vi "GoToKick.vi"(1 "goleiro?":bool, 3 "balls":T3[](array[typedef]), 4 "Robot in in":T4, 5 "atacando contra?":bool, 6 "Field Size in":T2, 7 "Target":dbl[](array[numeric]), 8 "Defender":bool, 9 "D ball - robot":dbl, 10 "AI Parameters":T1={"GotoKick"={"Dist do cone a frente"=150.0, "attacker farback"=1500.0, "Perto"=300.0, "min dist to kick"=150.0, "kick eps"=0.05, "Time to transition"=0.0}, "Attacker"={"CC chute"=0.09, "CC passe"=0.045, "Kick Force"=100.0, "D ball-robot Kick"=200.0, "D ball-robot Pass"=0.3}, "Defender"={"D max"=1700.0, "Vel p/ robô av"=1000.0, "Kick Force"=100.0, "D atk-def"=0.0, "D farback"=0.0}, "Timeout"={"Field/v in x"=6.0, "Dist Robots"=300, "Dist up in y"=300}, "Pose Striker"={"dist"=200.0, "Numeric"=-4.0, "dist 2"=200.0}, "Dist Stop"=300.0, "Distance when ball out"=200, "D central gap "=150.0, "T pass"=0.0, "Force ++"=0.0, "range kick"=0.0, "Chute alto"=TRUE, "Marcador novo"=TRUE} {"D central gap" format="%#_13g"; "Dist Stop" format="%#_13g"; "Pose Striker"."Numeric" format="%#_13g"; "Defender"."Kick Force" format="%#_13g"; "Defender"."Vel p/ robô av" format="%#_13g"; "Attacker"."D ball-robot Kick" format="%#_13g"; "Attacker"."Kick Force" format="%#_13g"; "Attacker"."CC passe" format="%#_13g"; "Attacker"."CC chute" format="%#_13g"; "GotoKick"."kick eps" format="%#_13g"; "GotoKick"."min dist to kick" format="%#_13g"; "GotoKick"."Perto" format="%#_13g"; "GotoKick"."attacker farback" format="%#_13g"; "GotoKick"."Dist do cone a frente" format="%#_13g"}, 11 "Cone de chute":dbl=0.09 format="%#_13g", 13 "Passe":bool, 18 "Kick Force":dbl=5.0 format="%#_13g", 19 "IA State Input in":T7) -> (0 "Current States":T6, 12 "Next State":T6, 14 "Robot out":T4, 17 "kick error":dbl)   [LabVIEW 2017]
uses:
  Core/AI Input.ctl
  Core/AI Robot.ctl
  Functions Enum.ctl
  AttackerStates.ctl
  Core/AI Ball.ctl
  Core/Field Size.ctl
  Core/AI Judge.ctl
  Command Enum.ctl
  Util/Events/Events.ctl
  AI Parameters.ctl
  <vilib>/Analysis/_algsub.llb/Real Vector Norm.vi
  <vilib>/Analysis/baseanly.llb/Real Dot Product.vi
  <vilib>/Analysis/coordinate.llb/2D Cartesian Coordinate Rotation (Scalar).vi
  <vilib>/Analysis/NI_AALPro.lvlib
  <vilib>/Analysis/NI_AALBase.lvlib
panel:
  out "Elapsed Time (s)":dbl
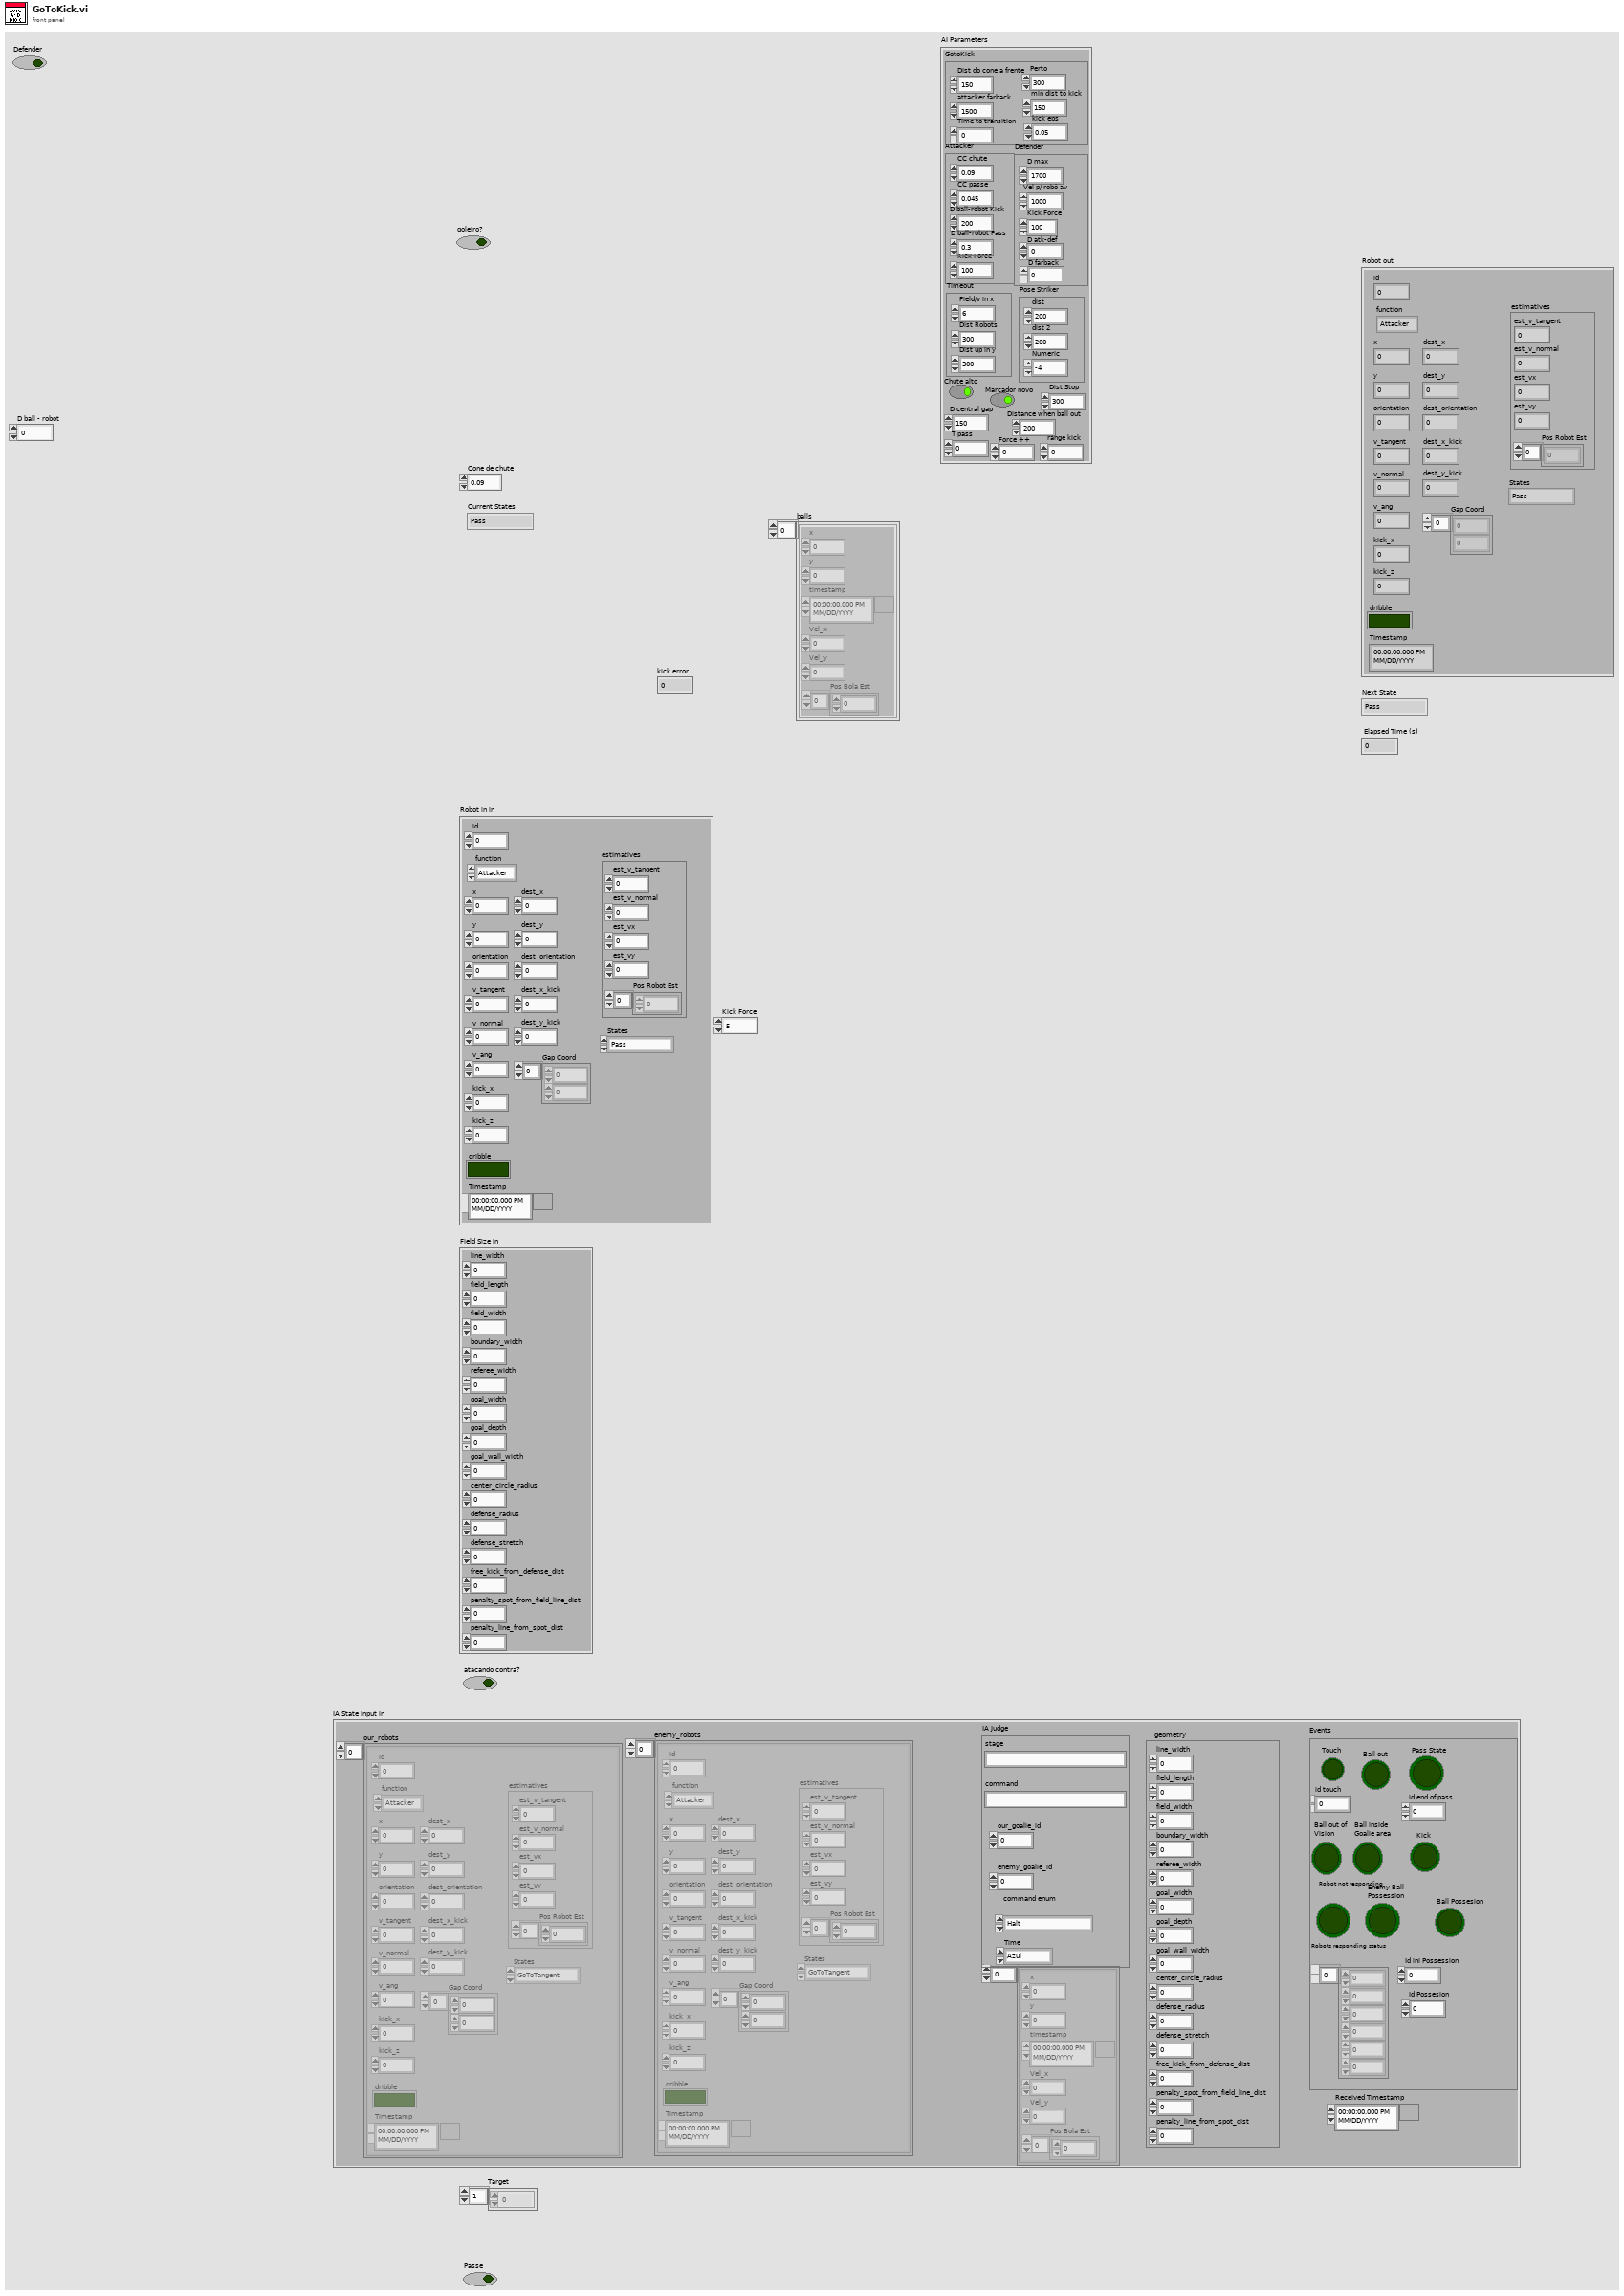
[diagram p1: front panel]
types:
  T1 = typedef "AI Parameters.ctl" = cluster{"GotoKick":cluster{"Dist do cone a frente":dbl, "attacker farback":dbl, "Perto":dbl, "min dist to kick":dbl, "kick eps":dbl, "Time to transition":dbl}, "Attacker":cluster{"CC chute":dbl, "CC passe":dbl, "Kick Force":dbl, "D ball-robot Kick":dbl, "D ball-robot Pass":dbl}, "Defender":cluster{"D max":dbl, "Vel p/ robô av":dbl, "Kick Force":dbl, "D atk-def":dbl, "D farback":dbl}, "Timeout":cluster{"Field/v in x":dbl, "Dist Robots":u32, "Dist up in y":u32}, "Pose Striker":cluster{"dist":dbl, "Numeric":dbl, "dist 2":dbl}, "Dist Stop":dbl, "Distance when ball out":i32, "D central gap ":dbl, "T pass":dbl, "Force ++":dbl, "range kick":dbl, "Chute alto":bool, "Marcador novo":bool}
  T2 = typedef "Field Size.ctl" = cluster{"line_width":u32, "field_length":u32, "field_width":u32, "boundary_width":u32, "referee_width":u32, "goal_width":u32, "goal_depth":u32, "goal_wall_width":u32, "center_circle_radius":u32, "defense_radius":u32, "defense_stretch":u32, "free_kick_from_defense_dist":u32, "penalty_spot_from_field_line_dist":u32, "penalty_line_from_spot_dist":u32}
  T3 = typedef "AI Ball.ctl" = cluster{"x":dbl, "y":dbl, "timestamp":timestamp, "Vel_x":dbl, "Vel_y":dbl, "Pos Bola Est":dbl[]}
  T4 = typedef "AI Robot.ctl" = cluster{"id":u32, "function":T5, "x":dbl, "y":dbl, "orientation":dbl, "v_tangent":dbl, "v_normal":dbl, "v_ang":dbl, "kick_x":dbl, "kick_z":dbl, "dribble":bool, "Timestamp":timestamp, "dest_x":dbl, "dest_y":dbl, "dest_orientation":dbl, "estimatives":cluster{"est_v_tangent":dbl, "est_v_normal":dbl, "est_vx":dbl, "est_vy":dbl, "Pos Robot Est":dbl[]}, "dest_x_kick":dbl, "dest_y_kick":dbl, "Gap Coord":dbl[], "States":T6}
  T5 = typedef "Functions Enum.ctl" = enum16{"Attacker", "Goalie", "Defender", "Striker", "Goto 0", "Dummy", "Kicker", "ZigZag"}
  T6 = typedef "AttackerStates.ctl" = enum16{"Pass", "GoToTangent", "BallGetting", "GoToKick", ""}
  T7 = typedef "AI Input.ctl" = cluster{"our_robots":T4[], "enemy_robots":T4[], "balls":T3[], "geometry":T2, "IA Judge":T8, "Received Timestamp":timestamp, "Events":T10}
  T8 = typedef "AI Judge.ctl" = cluster{"stage":string, "command":string, "our_goalie_id":dbl, "enemy_goalie_id":dbl, "command enum":T9, "Time":enum16{"Azul", "Amarelo"}}
  T9 = typedef "Command Enum.ctl" = enum16{"Halt", "Stop", "Force Start", "PKA Normal Start", "Prepare Kickoff Ally", "PKE Normal Start", "Prepare Kickoff Enemy", "Prepare Penalty Ally", "PPA Normal Start", "Prepare Penalty Enemy", "PPE Normal Start", "Direct Free Enemy", "Direct Free Ally", "Indirect Free Enemy", "Indirect Free Ally", "Timeout Enemy", "Timeout Ally", "Goal Enemy", "Goal Ally", "Ball Placement Enemy", "Ball Placement Ally", "Normal Half Time", "Extra Time Break", "Extra Half Time", "None", "Post Game"}
  T10 = typedef "Events.ctl" = cluster{"Touch":bool, "Ball out":bool, "id touch":dbl, "Ball out of \nVision":bool, "Ball inside \nGoalie area":bool, "Robot not responding":bool, "Robots responding status":dbl[], "Enemy Ball \nPossession":bool, "Pass State":bool, "id end of pass":dbl, "Kick":bool, "Id ini Possession":dbl, "Ball Possesion":bool, "Id Possesion":dbl}
  T11 = cluster{"Dist do cone a frente":dbl, "attacker farback":dbl, "Perto":dbl, "min dist to kick":dbl, "kick eps":dbl, "Time to transition":dbl}
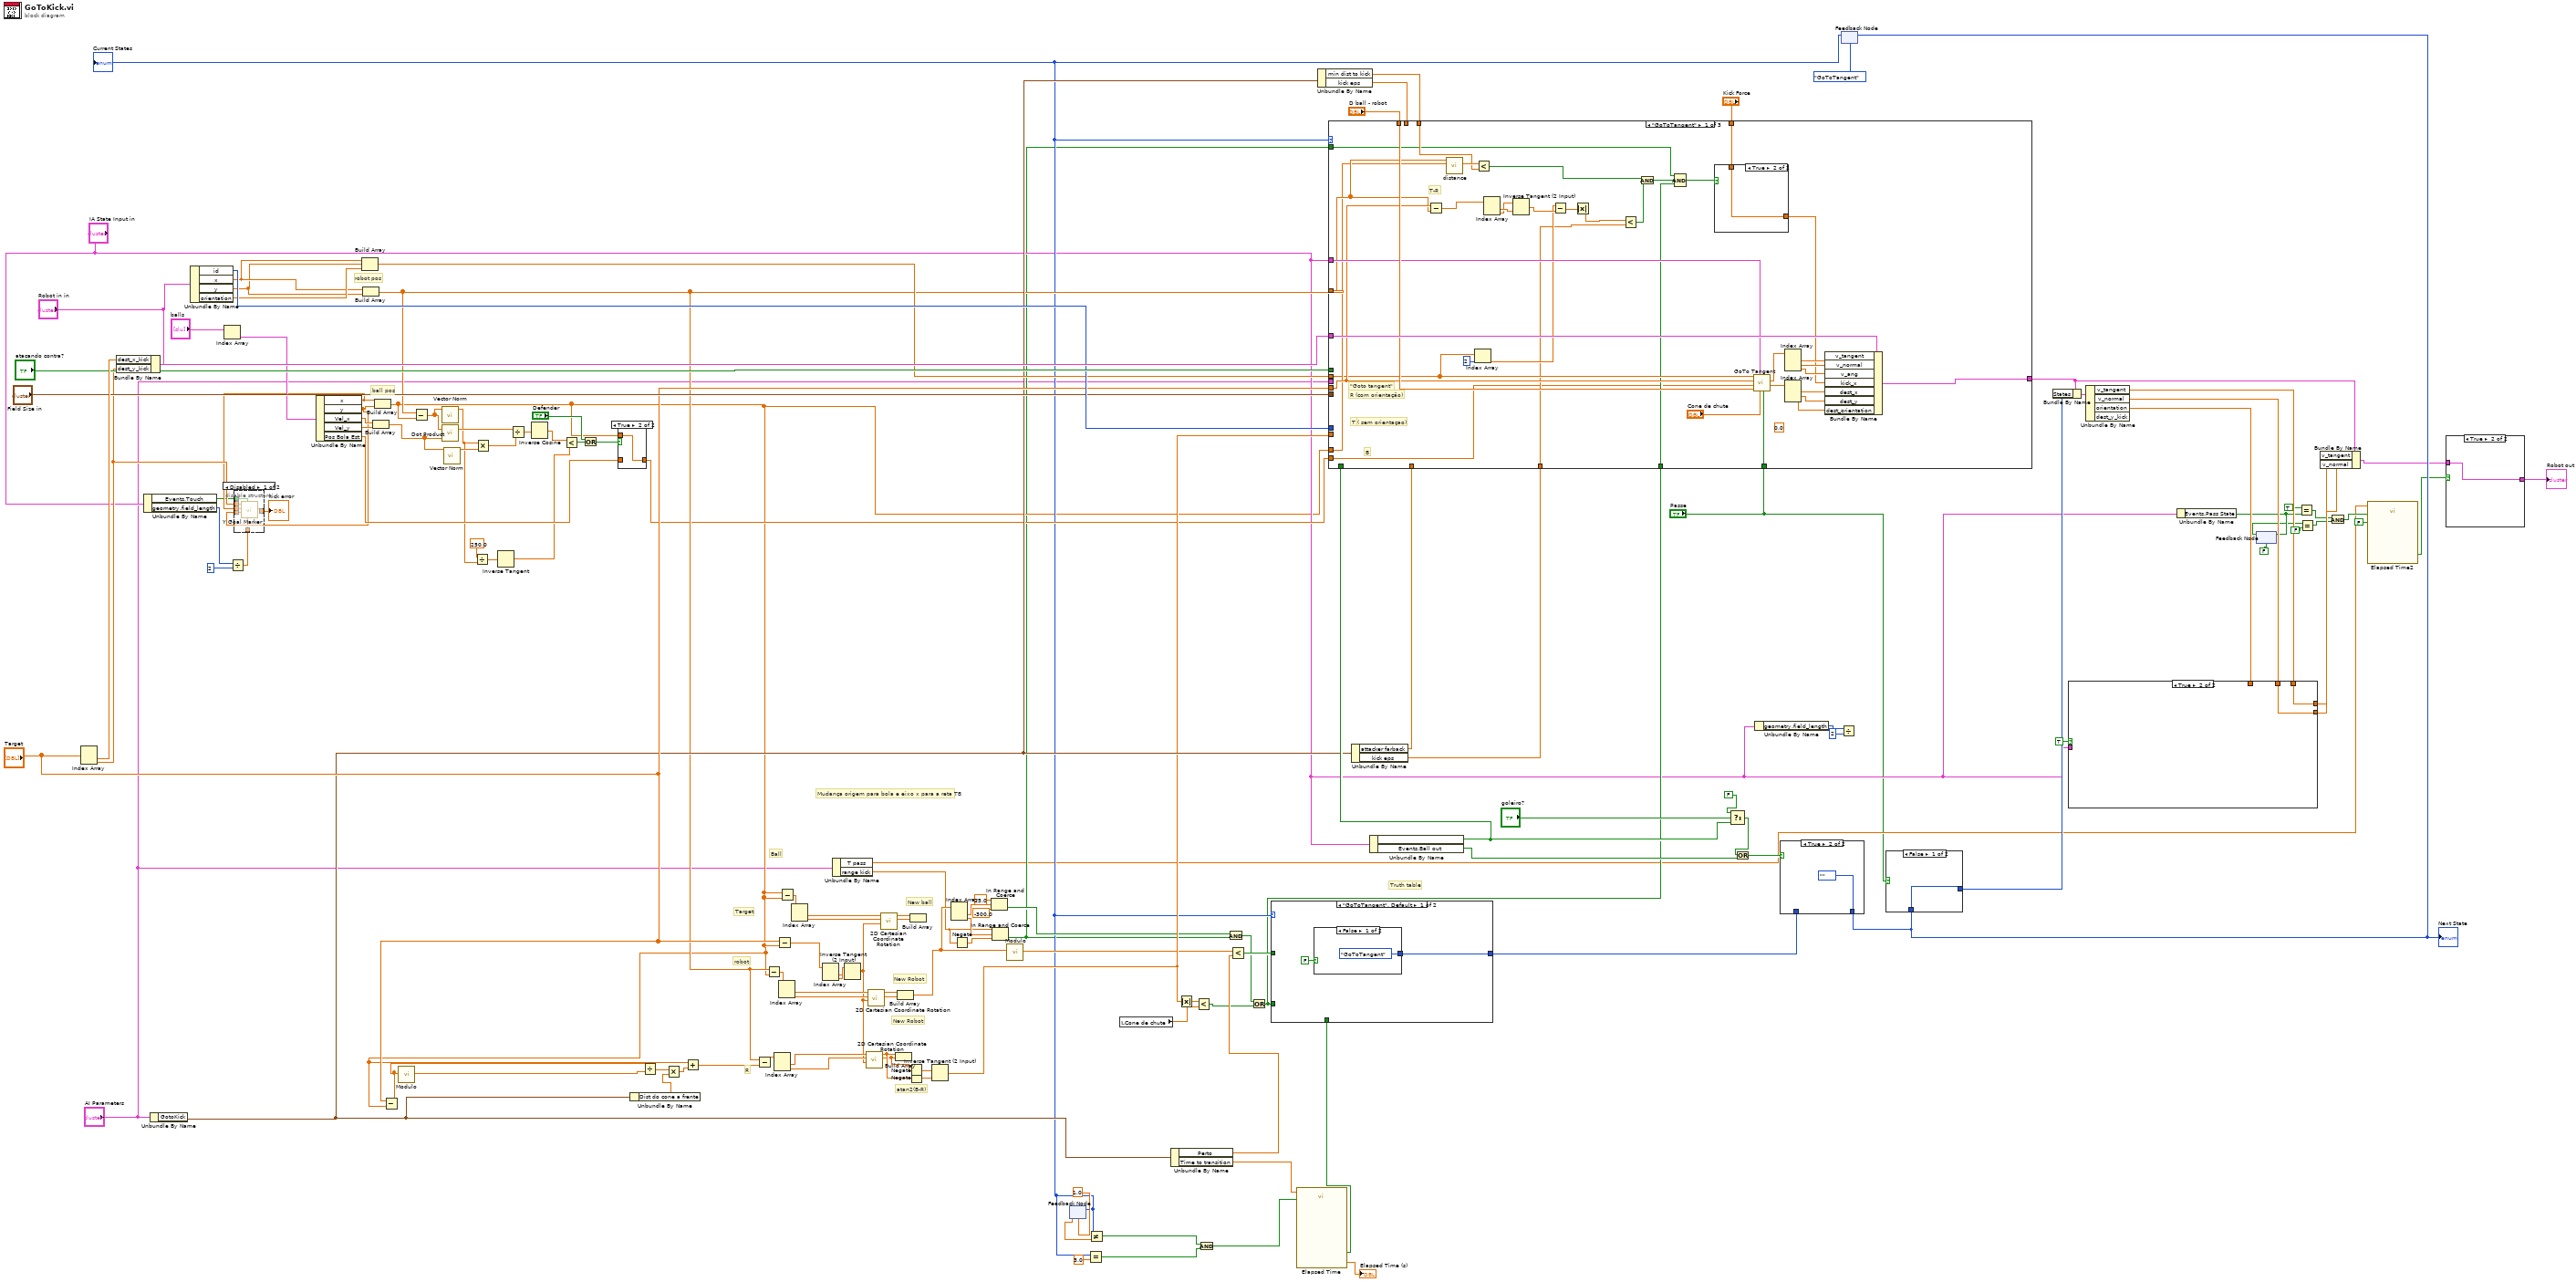
[diagram p0: block diagram]
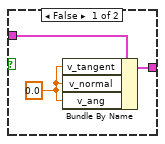
[diagram p3: hidden frame]
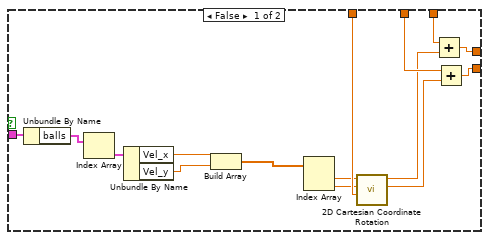
[diagram p4: hidden frame]
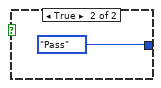
[diagram p6: hidden frame]
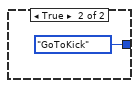
[diagram p7: hidden frame]
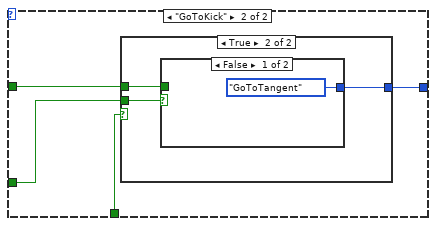
[diagram p8: hidden frame]
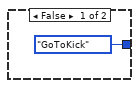
[diagram p9: hidden frame]
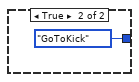
[diagram p10: hidden frame]
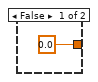
[diagram p12: hidden frame]
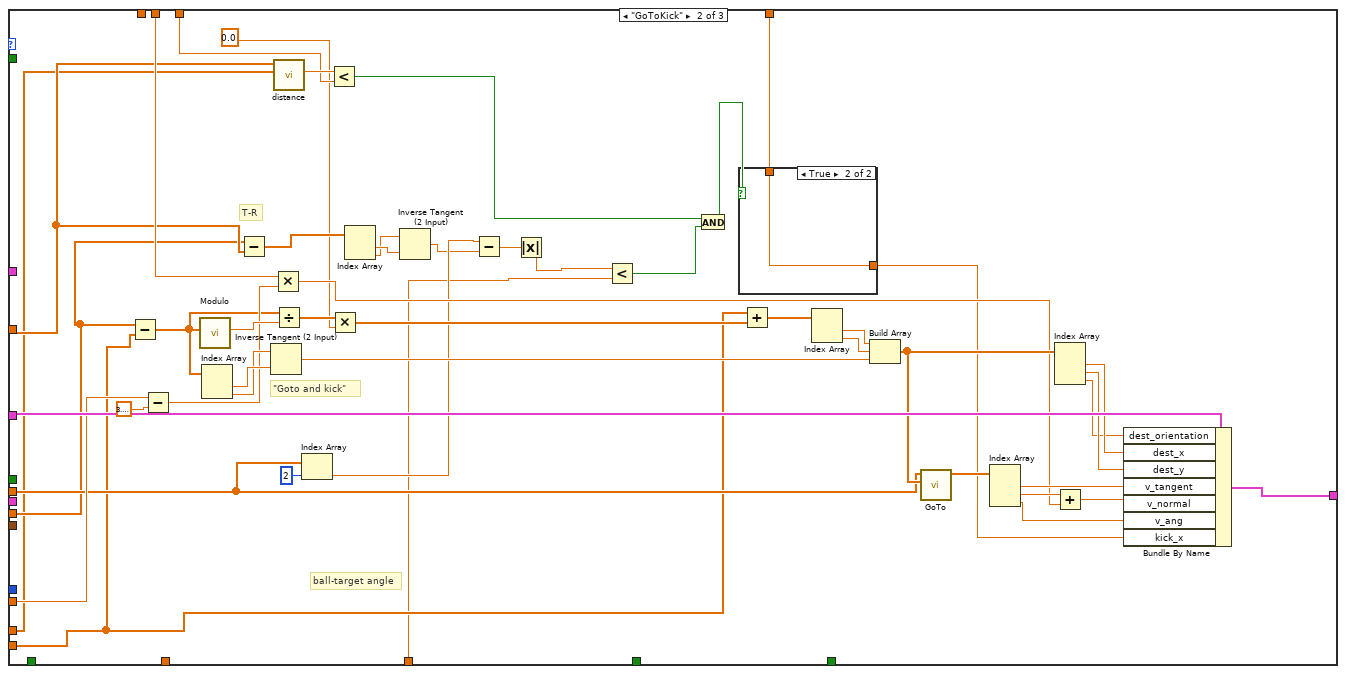
[diagram p13: hidden frame]
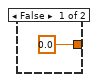
[diagram p14: hidden frame]
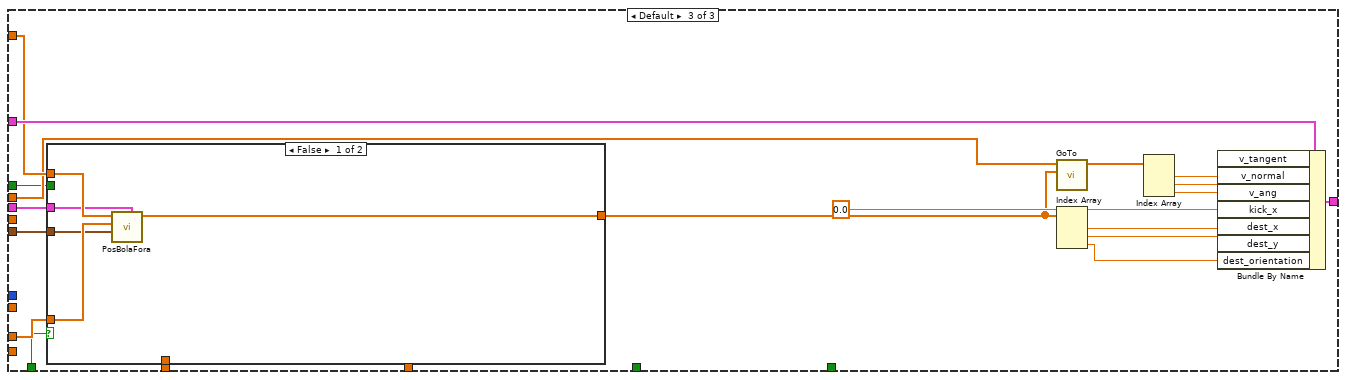
[diagram p15: hidden frame]
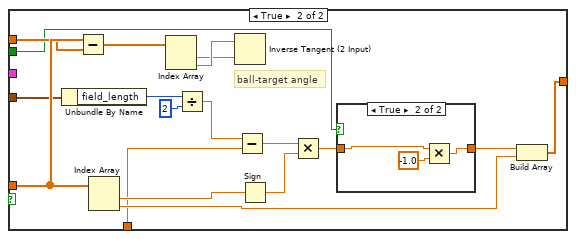
[diagram p16: hidden frame]
diagram:
  # "New ball"
  # "robot"
  # "atan2(B-R)"
  # "New Robot"
  # "New Robot"
  # "R"
  # "Ball"
  # "Target"
  # "Mudança origem para bola e eixo x para a reta TB"
  # "Truth table"
  # "robot pos"
  # "ball pos"
  n1 = Index Array(array="Target") -> (element #1=w139:dbl, element #2=w34:dbl)  [unwired: 2 in]
  n2 = Bundle By Name(cluster="Robot in in", "dest_x_kick"=w139, "dest_y_kick"=w34) -> (w135:T4)
  n3 = Unbundle By Name("IA State Input in") -> ("Events.Touch"=w30:bool, "geometry.field_length"=w29:u32)
  n4 = Unbundle By Name("AI Parameters") -> ("GotoKick"=w80:T11)
  n5 = Unbundle By Name("Robot in in") -> ("id"=w110:u32, "x"=w74:dbl, "y"=w73:dbl, "orientation"=w101:dbl)
  n6 = Index Array(array="balls") -> (element=w99:T3)  [unwired: 1 in]
  n7 = Divide(x=w29, y=u32 2) -> (x/y=w27:dbl)
  n8 = Unbundle By Name(w99) -> ("x"=w33:dbl, "y"=w32:dbl, "Vel_x"=w56:dbl, "Vel_y"=w55:dbl, "Pos Bola Est"=w47:dbl[])
  n9 = disable-structure shown="Disabled" {
    disable-tunnel: w34 -> [w145 _]
    disable-tunnel: w33 -> [w144 _]
    disable-tunnel: w32 -> [w143 _]
    disable-tunnel: w30 -> [w142 _]
    disable-tunnel: w27 -> [w141 _]
    disable-tunnel: [w140 _] -> w26
    frame Disabled {
      n10 = call "Y Goal Marker.vi"("goal x"=w141, "Touch"=w142, "ball y"=w143, "ball x"=w144, "dest_y_kick"=w145) -> ("kick error"=w140:dbl)  [unwired: 5 in, 1 out]
    }
    frame Enabled {
    }
  }
  "kick error" <- w26
  n11 = Build Array(w74, w73, w101) -> (w100:dbl[])
  n12 = Build Array(w74, w73) -> (w57:dbl[])
  n13 = Build Array(w56, w55) -> (w53:dbl[])
  n14 = Build Array(w33, w32) -> (w20:dbl[])
  n15 = Subtract(x="Target", y=w20) -> (x-y=w129:dbl[])
  n16 = call "Modulo.vi"("2D vector"=w129) -> ("Modulo"=w128:dbl)  [unwired: 10 in]
  n17 = Subtract(x=w57, y=w20) -> (x-y=w54:dbl[])
  n18 = call-poly <vilib>:"Dot Product.vi"("Y Vector"=w53, "X Vector"=w54) -> ("X * Y"=w50:dbl)  [unwired: 1 out]
  n19 = call-poly <vilib>:"Vector Norm.vi"("Input Vector"=w54) -> ("norm"=w44:dbl)  [unwired: 9 in, 1 out]
  n20 = call-poly <vilib>:"Vector Norm.vi"("Input Vector"=w53) -> ("norm"=w52:dbl)  [unwired: 9 in, 1 out]
  n21 = Divide(x=250.0, y=w44) -> (x/y=w45:dbl)
  n22 = Multiply(x=w44, y=w52) -> (x*y=w51:dbl)
  n23 = Inverse Tangent(1:w45) -> (0:w42:dbl)
  n24 = Divide(x=w50, y=w51) -> (x/y=w49:dbl)
  n25 = Inverse Cosine(1:w49) -> (0:w48:dbl)
  n26 = Less?(x=w48, y=w42) -> (x < y?=w22:bool)
  n27 = Or(x="Defender", y=w22) -> (x .or. y?=w23:bool)
  n28 = case shown="True" w23 {
    tunnel: w47 -> [w146 _]
    tunnel: [w146 w147] -> w46
    tunnel: w20 -> [_ w147]
    frame False {
    }
    frame True {
    }
  }
  n29 = Unbundle By Name(w80) -> ("Dist do cone a frente"=w86:dbl)
  n30 = Divide(x=w129, y=w128) -> (x/y=w127:dbl[])
  n31 = Multiply(x=w127, y=w86) -> (x*y=w126:dbl[])
  n32 = Add(x=w20, y=w126) -> (x+y=w130:dbl[])
  n33 = Subtract(x=w57, y=w130) -> (x-y=w131:dbl[])
  n34 = Subtract(x=w57, y=w20) -> (x-y=w104:dbl[])
  n35 = Index Array(array=w131) -> (element #1=w132:dbl, element #2=w133:dbl)  [unwired: 2 in]
  n36 = Subtract(x="Target", y=w20) -> (x-y=w105:dbl[])
  n37 = Index Array(array=w104) -> (element #1=w102:dbl, element #2=w103:dbl)  [unwired: 2 in]
  n38 = Subtract(x=w20, y=w20) -> (x-y=w70:dbl[])
  n39 = Index Array(array=w70) -> (element #1=w68:dbl, element #2=w69:dbl)  [unwired: 2 in]
  n40 = Index Array(array=w105) -> (element #1=w106:dbl, element #2=w107:dbl)  [unwired: 2 in]
  n41 = Unbundle By Name("AI Parameters") -> ("T pass"=w2:dbl, "range kick"=w3:dbl)
  n42 = Inverse Tangent (2 Input)(1:w106, 2:w107) -> (0:w67:dbl)
  n43 = call-poly <vilib>:"2D Cartesian Coordinate Rotation.vi"("theta"=w67, "y"=w133, "x"=w132) -> ("y out"=w124:dbl, "x out"=w125:dbl)  [unwired: 6 in, 1 out]
  n44 = call-poly <vilib>:"2D Cartesian Coordinate Rotation.vi"("theta"=w67, "y"=w103, "x"=w102) -> ("y out"=w109:dbl, "x out"=w66:dbl)  [unwired: 6 in, 1 out]
  n45 = call-poly <vilib>:"2D Cartesian Coordinate Rotation.vi"("theta"=w67, "y"=w69, "x"=w68) -> ("y out"=w71:dbl, "x out"=w72:dbl)  [unwired: 6 in, 1 out]
  n46 = Build Array(w125, w124) -> ()  [unwired: 1 out]
  n47 = Build Array(w66, w109) -> (w65:dbl[])
  n48 = Negate(x=w124) -> (-x=w122:dbl)
  n49 = Negate(x=w125) -> (-x=w123:dbl)
  n50 = Build Array(w72, w71) -> ()  [unwired: 1 out]
  n51 = Inverse Tangent (2 Input)(1:w123, 2:w122) -> (0:w78:dbl)
  n52 = Index Array(array=w65) -> (element #1=w64:dbl, element #2=w63:dbl)  [unwired: 2 in]
  n53 = Negate(x=w3) -> (-x=w4:dbl)
  n54 = In Range and Coerce(upper limit=25.0, x=w64, lower limit=-300.0) -> (In Range?=w60:bool)  [unwired: 1 out]
  n55 = In Range and Coerce(upper limit=w3, x=w63, lower limit=w4) -> (In Range?=w6:bool)  [unwired: 1 out]
  n56 = call "Modulo.vi"("2D vector"=w65) -> ("Modulo"=w77:dbl)  [unwired: 10 in]
  n57 = feedback #1(1.0 ("Current State")) -> (w116:dbl)
  n58 = local read "Cone de chute"() -> (w25:dbl)
  n59 = Unbundle By Name(w80) -> ("Perto"=w76:dbl, "Time to transition"=w82:dbl)
  n60 = Absolute Value(x=w78) -> (abs(x)=w79:dbl)
  n61 = Less?(x=w79, y=w25) -> (x < y?=w59:bool)
  n62 = And(x=w60, y=w6) -> (x .and. y?=w58:bool)
  n63 = Less?(x=w77, y=w76) -> (x < y?=w75:bool)
  n64 = Or(x=w58, y=w59) -> (x .or. y?=w39:bool)
  n65 = Unbundle By Name(w80) -> ("min dist to kick"=w84:dbl, "kick eps"=w83:dbl)
  n66 = Unbundle By Name(w80) -> ("attacker farback"=w85:dbl, "kick eps"=w35:dbl)
  n67 = Unbundle By Name("IA State Input in") -> ("Events.Ball inside \nGoalie area"=w88:bool, "Events.Ball out"=w120:bool)
  n68 = Select(t=FALSE, s="goleiro?", f=w88) -> (s? t:f=w87:bool)
  n69 = Or(x=w87, y=w120) -> (x .or. y?=w121:bool)
  n70 = Unbundle By Name("IA State Input in") -> ("geometry.field_length"=w37:u32)
  n71 = Divide(x=w37, y=u32 2) -> ()  [unwired: 1 out]
  n72 = feedback #2(AttackerStates."GoToTangent" ("Next State")) -> (w41:T6)
  "Current States" <- w41
  n73 = feedback-in #1(w41) -> ()
  n74 = Equal?(x=w41, y=3.0) -> (x = y?=w113:bool)
  n75 = Not Equal?(x=w41, y=w116) -> (x != y?=w114:bool)
  n76 = And(x=w114, y=w113) -> (x .and. y?=w118:bool)
  n77 = call "Elapsed Time"("Time Target (s)"=w82, "Reset"=w118) -> ("Elapsed Time (s)"=→"Elapsed Time (s)":dbl, "Time has Elapsed"=w111:bool)  [unwired: 10 in, 6 out]
  n78 = case shown="\"GoToTangent\", Default" w41 {
    tunnel: [w149 w154] -> w136
    tunnel: w111 -> [_ w155]
    tunnel: w39 -> [_ w153]
    tunnel: w75 -> [_ w152]
    frame "GoToTangent", Default {
      n79 = case shown="False" FALSE {
        tunnel: [AttackerStates."GoToTangent" ("Next State") AttackerStates."GoToKick" ("Next State")] -> w149
        frame False {
        }
        frame True {
        }
      }
    }
    frame "GoToKick" {
      n80 = case shown="True" w155 {
        tunnel: [AttackerStates."GoToKick" ("Next State") w159] -> w154
        tunnel: w153 -> [_ w158]
        tunnel: w152 -> [_ w157]
        frame False {
        }
        frame True {
          n81 = case shown="False" w158 {
            tunnel: [AttackerStates."GoToTangent" ("Next State") AttackerStates."GoToKick" ("Next State")] -> w159
            tunnel: w157 -> [_ _]
            frame False {
            }
            frame True {
            }
          }
        }
      }
    }
  }
  n82 = case shown="\"GoToTangent\"" w41 {
    tunnel: [w191 w249 w270] -> w38
    tunnel: w135 -> [w192 w248 w269]
    tunnel: w100 -> [w172 w215 w263]
    tunnel: w57 -> [w176 w209 w265]
    tunnel: w20 -> [w175 w205 w266]
    tunnel: "Target" -> [w177 w208 _]
    tunnel: "Field Size in" -> [_ _ w264]
    tunnel: w110 -> [_ _ _]
    tunnel: w88 -> [_ _ w259]
    tunnel: "atacando contra?" -> [_ _ w258]
    tunnel: w78 -> [_ w229 _]
    tunnel: w85 -> [_ _ w253]
    tunnel: w84 -> [w174 w223 _]
    tunnel: w83 -> [_ w222 _]
    tunnel: "D ball - robot" -> [w189 _ _]
    tunnel: "AI Parameters" -> [_ _ w252]
    tunnel: "IA State Input in" -> [w188 _ _]
    tunnel: w46 -> [w164 w206 _]
    tunnel: "Kick Force" -> [w178 w204 _]
    tunnel: w39 -> [w168 _ _]
    tunnel: w35 -> [w166 w203 _]
    tunnel: w6 -> [w163 _ _]
    tunnel: "Passe" -> [w162 _ _]
    frame "GoToTangent" {
      (unwired) 0.0
      # "T-R"
      # "\"Goto tangent\""
      # "B"
      # "T"
      # "R ( sem orientaçao)"
      # "R (com orientação)"
      n83 = Subtract(x=w177, y=w176) -> (x-y=w184:dbl[])
      n84 = call "distance.vi"("target pos"=w175, "obj pos"=w176) -> ("sqrt(x)"=w187:dbl)  [unwired: 9 in]
      n85 = Index Array(array=w172, index=2) -> (element=w171:dbl)
      n86 = Less?(x=w187, y=w174) -> (x < y?=w183:bool)
      n87 = Index Array(array=w184) -> (element #1=w186:dbl, element #2=w185:dbl)  [unwired: 2 in]
      n88 = Inverse Tangent (2 Input)(1:w186, 2:w185) -> (0:w182:dbl)
      n89 = Subtract(x=w171, y=w182) -> (x-y=w181:dbl)
      n90 = Absolute Value(x=w181) -> (abs(x)=w179:dbl)
      n91 = Less?(x=w179, y=w166) -> (x < y?=w180:bool)
      n92 = And(x=w183, y=w180) -> (x .and. y?=w169:bool)
      n93 = Compound Arithmetic op=AND(w163, w169, w168) -> (w167:bool)
      n94 = case shown="True" w167 {
        tunnel: [0.0 w201] -> w170
        tunnel: w178 -> [_ w201]
        frame False {
        }
        frame True {
        }
      }
      n95 = call "GoTo Tangent.vi"("Passe"=w162, "Cone de chute"="Cone de chute", "IA State Input in"=w188, "distance between ball and robot"=w189, "Ball"=w164, "Target"=w177, "R"=w172) -> ("Destination"=w196:dbl[], "Output\nVelocity"=w197:dbl[])  [unwired: 3 in]
      n96 = Index Array(array=w197) -> (element #1=w199:dbl, element #2=w193:dbl, element #3=w198:dbl)  [unwired: 3 in]
      n97 = Index Array(array=w196) -> (element #1=w195:dbl, element #2=w194:dbl, element #3=w190:dbl)  [unwired: 3 in]
      n98 = Bundle By Name(cluster=w192, "v_tangent"=w199, "v_normal"=w193, "v_ang"=w198, "kick_x"=w170, "dest_x"=w195, "dest_y"=w194, "dest_orientation"=w190) -> (w191:T4)
    }
    frame "GoToKick" {
      # "T-R"
      # "ball-target angle"
      # "\"Goto and kick\""
      n99 = Subtract(x=w208, y=w206) -> (x-y=w219:dbl[])
      n100 = Subtract(x=w229, y=3.141592653589793) -> (x-y=w227:dbl)
      n101 = call "Modulo.vi"("2D vector"=w219) -> ("Modulo"=w236:dbl)  [unwired: 10 in]
      n102 = Index Array(array=w219) -> (element #1=w246:dbl, element #2=w245:dbl)  [unwired: 2 in]
      n103 = Subtract(x=w208, y=w209) -> (x-y=w218:dbl[])
      n104 = Inverse Tangent (2 Input)(1:w246, 2:w245) -> (0:w244:dbl)
      n105 = Multiply(x=w222, y=w227) -> (x*y=w230:dbl)
      n106 = call "distance.vi"("target pos"=w205, "obj pos"=w209) -> ("sqrt(x)"=w247:dbl)  [unwired: 9 in]
      n107 = Divide(x=w219, y=w236) -> (x/y=w237:dbl[])
      n108 = Index Array(array=w215, index=2) -> (element=w213:dbl)
      n109 = Less?(x=w247, y=w223) -> (x < y?=w217:bool)
      n110 = Multiply(x=w237, y=0.0) -> (x*y=w239:dbl[])
      n111 = Index Array(array=w218) -> (element #1=w221:dbl, element #2=w220:dbl)  [unwired: 2 in]
      n112 = Inverse Tangent (2 Input)(1:w221, 2:w220) -> (0:w212:dbl)
      n113 = Subtract(x=w213, y=w212) -> (x-y=w211:dbl)
      n114 = Absolute Value(x=w211) -> (abs(x)=w207:dbl)
      n115 = Less?(x=w207, y=w203) -> (x < y?=w210:bool)
      n116 = And(x=w217, y=w210) -> (x .and. y?=w216:bool)
      n117 = case shown="True" w216 {
        tunnel: [0.0 w251] -> w226
        tunnel: w204 -> [_ w251]
        frame False {
        }
        frame True {
        }
      }
      n118 = Add(x=w206, y=w239) -> (x+y=w238:dbl[])
      n119 = Index Array(array=w238) -> (element #1=w243:dbl, element #2=w242:dbl)  [unwired: 2 in]
      n120 = Build Array(w243, w242, w244) -> (w234:dbl[])
      n121 = call "GoTo.vi"("Target"=w234, "Position"=w215) -> ("Output\nVelocity"=w241:dbl[])  [unwired: 8 in, 1 out]
      n122 = Index Array(array=w241) -> (element #1=w240:dbl, element #2=w232:dbl, element #3=w225:dbl)  [unwired: 3 in]
      n123 = Index Array(array=w234) -> (element #1=w235:dbl, element #2=w233:dbl, element #3=w224:dbl)  [unwired: 3 in]
      n124 = Add(x=w232, y=w230) -> (x+y=w231:dbl)
      n125 = Bundle By Name(cluster=w248, "dest_orientation"=w224, "dest_x"=w235, "dest_y"=w233, "v_tangent"=w240, "v_normal"=w231, "v_ang"=w225, "kick_x"=w226) -> (w249:T4)
    }
    frame Default {
      n126 = case shown="False" w259 {
        tunnel: w266 -> [w275 w287]
        tunnel: w265 -> [w274 w285]
        tunnel: w264 -> [w273 w286]
        tunnel: [w272 w292] -> w261
        tunnel: w258 -> [_ w281]
        tunnel: w253 -> [_ w276]
        tunnel: w252 -> [w271 _]
        frame False {
          n127 = call "PosBolaFora.vi"("AI Parameters"=w271, "Field Size in"=w273, "Position da bola"=w275, "Position do robot"=w274) -> ("Target"=w272:dbl[])  [unwired: 7 in]
        }
        frame True {
          # "ball-target angle"
          n128 = Unbundle By Name(w286) -> ("field_length"=w284:u32)
          n129 = Subtract(x=w287, y=w285) -> (x-y=w290:dbl[])
          n130 = Index Array(array=w287) -> (element #1=w280:dbl, element #2=w293:dbl)  [unwired: 2 in]
          n131 = Index Array(array=w290) -> (element #1=w288:dbl, element #2=w289:dbl)  [unwired: 2 in]
          n132 = Divide(x=w284, y=u32 2) -> (x/y=w282:dbl)
          n133 = Inverse Tangent (2 Input)(1:w288, 2:w289) -> ()  [unwired: 1 out]
          n134 = Subtract(x=w282, y=w276) -> (x-y=w279:dbl)
          n135 = Sign(1:w280) -> (0:w278:dbl)
          n136 = Multiply(x=w279, y=w278) -> (x*y=w277:dbl)
          n137 = case shown="True" w281 {
            tunnel: w277 -> [w294 w297]
            tunnel: [w294 w296] -> w291
            frame False {
            }
            frame True {
              n138 = Multiply(x=w297, y=-1.0) -> (x*y=w296:dbl)
            }
          }
          n139 = Build Array(w291, w293) -> (w292:dbl[])
        }
      }
      n140 = call "GoTo.vi"("Target"=w261, "Position"=w263) -> ("Output\nVelocity"=w262:dbl[])  [unwired: 8 in, 1 out]
      n141 = Index Array(array=w261) -> (element #1=w260:dbl, element #2=w255:dbl, element #3=w254:dbl)  [unwired: 3 in]
      n142 = Index Array(array=w262) -> (element #1=w267:dbl, element #2=w257:dbl, element #3=w256:dbl)  [unwired: 3 in]
      n143 = Bundle By Name(cluster=w269, "v_tangent"=w267, "v_normal"=w257, "v_ang"=w256, "kick_x"=0.0, "dest_x"=w260, "dest_y"=w255, "dest_orientation"=w254) -> (w270:T4)
    }
  }
  n144 = case shown="True" w121 {
    tunnel: [w298 AttackerStates."" ("Next State")] -> w98
    tunnel: w136 -> [w298 _]
    frame False {
    }
    frame True {
    }
  }
  "Next State" <- w98
  n145 = feedback-in #2(w98) -> ()
  n146 = case shown="False" "Passe" {
    tunnel: w98 -> [w300 _]
    tunnel: [w300 AttackerStates."Pass" ("Next State")] -> w137
    frame False {
    }
    frame True {
    }
  }
  n147 = Bundle By Name(cluster=w38, "States"=w137) -> (w96:T4)
  n148 = Unbundle By Name(w96) -> ("v_tangent"=w94:dbl, "v_normal"=w93:dbl, "orientation"=w95:dbl)  [unwired: 1 out]
  n149 = case shown="True" TRUE {
    tunnel: w95 -> [w316 _]
    tunnel: w94 -> [w315 w318]
    tunnel: w93 -> [w314 w317]
    tunnel: [w313 w317] -> w92
    tunnel: [w312 w318] -> w91
    tunnel: "IA State Input in" -> [w311 _]
    frame False {
      n150 = Unbundle By Name(w311) -> ("balls"=w310:T3[])
      n151 = Index Array(array=w310) -> (element=w309:T3)  [unwired: 1 in]
      n152 = Unbundle By Name(w309) -> ("Vel_x"=w305:dbl, "Vel_y"=w304:dbl)
      n153 = Build Array(w305, w304) -> (w306:dbl[])
      n154 = Index Array(array=w306) -> (element #1=w308:dbl, element #2=w307:dbl)  [unwired: 2 in]
      n155 = call-poly <vilib>:"2D Cartesian Coordinate Rotation.vi"("theta"=w316, "y"=w307, "x"=w308) -> ("y out"=w302:dbl, "x out"=w303:dbl)  [unwired: 6 in, 1 out]
      n156 = Add(x=w315, y=w303) -> (x+y=w312:dbl)
      n157 = Add(x=w314, y=w302) -> (x+y=w313:dbl)
    }
    frame True {
    }
  }
  n158 = Unbundle By Name("IA State Input in") -> ("Events.Pass State"=w14:bool)
  n159 = feedback-in #3(w14) -> ()
  n160 = feedback #3(FALSE ("Pass State")) -> (w12:bool)
  n161 = Equal?(x=TRUE, y=w14) -> (x = y?=w9:bool)
  n162 = Equal?(x=w12, y=FALSE) -> (x = y?=w8:bool)
  n163 = Bundle By Name(cluster=w38, "v_tangent"=w91, "v_normal"=w92) -> (w18:T4)
  n164 = And(x=w9, y=w8) -> (x .and. y?=w7:bool)
  n165 = call "Elapsed Time2"("Time Target (s)"=w2, "Reset"=w7, "Auto Reset"=FALSE) -> ("Time has Elapsed"=w15:bool)  [unwired: 9 in, 7 out]
  n166 = case shown="True" w15 {
    tunnel: w18 -> [w321 w322]
    tunnel: [w320 w322] -> w17
    frame False {
      w319 = 0.0
      n167 = Bundle By Name(cluster=w321, "v_tangent"=w319, "v_normal"=w319, "v_ang"=w319) -> (w320:T4)
    }
    frame True {
    }
  }
  "Robot out" <- w17
